vi "Main.vi"   [LabVIEW 2020, in "OOP.lvlib"]
uses:
  OOP.lvlib
  Driver/Driver.lvclass
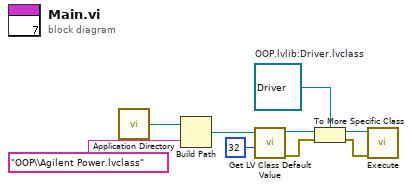
[diagram p0: block diagram]
diagram:
  w4 = refnum<class "Driver.lvclass"> refnum  # OOP.lvlib:Driver.lvclass
  n1 = call <vilib>:"Application Directory.vi"() -> ("Application Directory"=w9:path)
  n2 = Build Path(base path=w9, name or relative path="OOP\\Agilent Power.lvclass") -> (appended path=w7:path)
  n3 = call <vilib>:"Get LV Class Default Value.vi"("options"=u32 32, "class path"=w7) -> ("error out"=w2:errorcluster, "object"=w5:refnum<class>)  [unwired: 8 in]
  n4 = To More Specific Class(target class=w4, reference=w5, error in=w2) -> (specific class reference=w3:refnum<class "Driver.lvclass">, error out=w1:errorcluster)
  n5 = call-dynamic "Execute.vi"("error in (no error)"=w1, "Driver in"=w3) -> ()  [unwired: 8 in, 2 out]
